vi "Write configuration.vi"(8 "error in (no error)":errorcluster, 10 "configuration":refnum<class "CEF_serializable configuration.lvclass">, 11 "Thermo Instrument in":refnum<class "Thermo Instrument.lvclass">) -> (0 "error out":errorcluster, 3 "Thermo Instrument out":refnum<class "Thermo Instrument.lvclass">)   [LabVIEW 2025, in "Thermo.lvlib" / "Thermo Instrument.lvclass"]
uses:
  Thermo Instrument.lvclass
  Users/Public/Documents/Sandia National Labs/TSS Plugin/CEF.lvlibp/serializable configuration/CEF_serializable configuration.lvclass
  Thermo configuration/Thermo configuration.lvclass
  Thermo Instrument.lvclass/Thermo Instrument.ctl
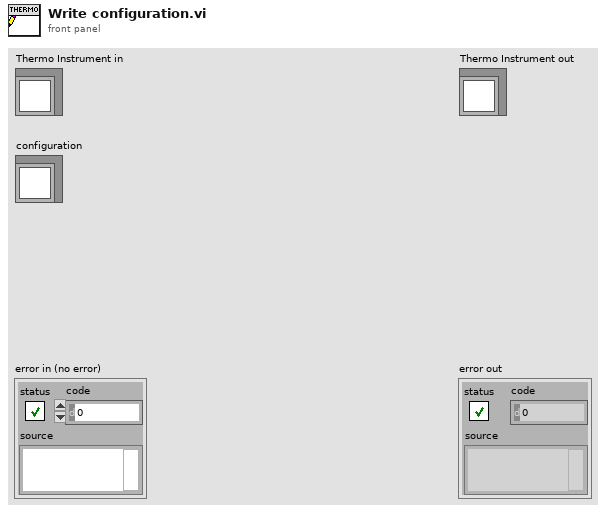
[diagram p1: front panel]
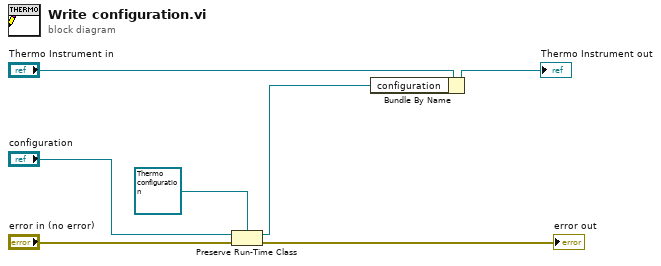
[diagram p0: block diagram]
diagram:
  n1 = Preserve Run-Time Class(object in="configuration", error in="error in (no error)", 2:refnum<class "Thermo configuration.lvclass"> refnum ("DMM.lvlib:DMM configuration.lvclass")) -> (object out=w2:refnum<class "Thermo configuration.lvclass">, error out=→"error out":errorcluster)
  n2 = Bundle By Name(cluster="Thermo Instrument in", "configuration"=w2) -> (→"Thermo Instrument out":refnum<class "Thermo Instrument.lvclass">)
